vi "Write shm info.vi"(8 "error in (no error)":errorcluster, 10 "shm info":T1, 11 "Shared Memory runtime in":refnum<class "Shared Memory runtime.lvclass">) -> (0 "error out":errorcluster, 3 "Shared Memory runtime out":refnum<class "Shared Memory runtime.lvclass">)   [LabVIEW 2013, in "Shared Memory runtime.lvclass"]
uses:
  Shared Memory runtime.lvclass
  controls/shm info.ctl
  <vilib>/NI/Shared Memory Library/Classes/Shared Memory/Public/Controls/reference.ctl
  <vilib>/NI/Shared Memory Library/Classes/Shared Memory/Shared Memory.lvclass
  controls/shm info ptrs.ctl
  Shared Memory runtime.lvclass/Shared Memory runtime.ctl
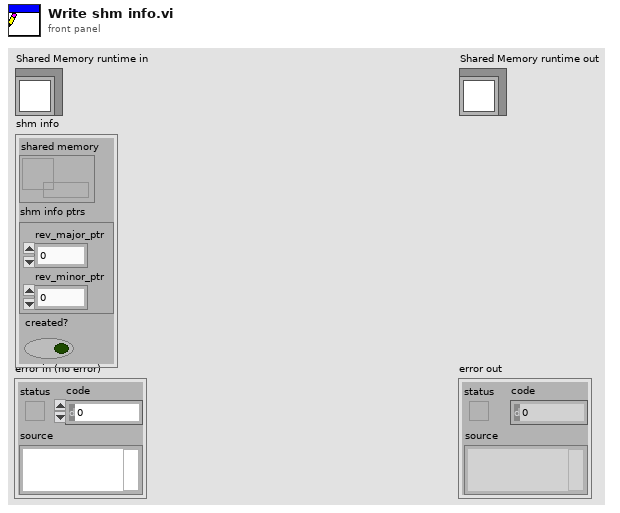
[diagram p1: front panel]
types:
  T1 = typedef "Shared Memory runtime.lvclass/shm info.ctl" = cluster{"shared memory":T2, "shm info ptrs":T3, "created?":bool}
  T2 = typedef "Shared Memory.lvlib/Shared Memory.lvclass/reference.ctl" = refnum<data-value>
  T3 = typedef "Shared Memory runtime.lvclass/shm info ptrs.ctl" = cluster{"rev_major_ptr":u64, "rev_minor_ptr":u64}
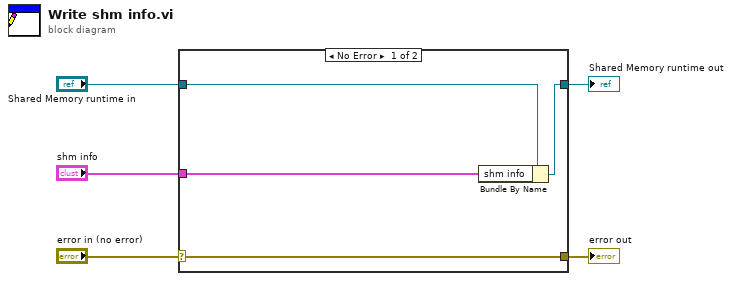
[diagram p0: block diagram]
diagram:
  n1 = case shown="No Error" "error in (no error)" {
    selector: "error in (no error)" -> [w9 w10]
    tunnel: [w9 w10] -> w4
    tunnel: [w7 w11] -> w2
    tunnel: "Shared Memory runtime in" -> [w8 w11]
    tunnel: "shm info" -> [w6 _]
    frame No Error {
      n2 = Bundle By Name(cluster=w8, "shm info"=w6) -> (w7:refnum<class "Shared Memory runtime.lvclass">)
    }
    frame Error {
    }
  }
  "error out" <- w4
  "Shared Memory runtime out" <- w2
